vi "Exc time Result.vi"(11 "SubVI":dbl[](array[numeric])) -> (3 "Pos":i32, 5 "Tip":string, 7 "Status":bool)   [LabVIEW 2014]
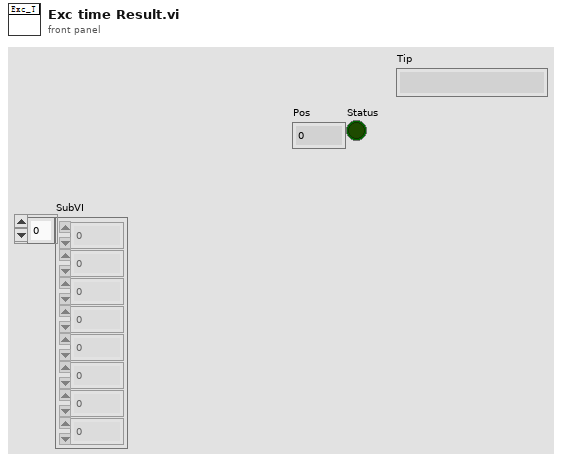
[diagram p1: front panel]
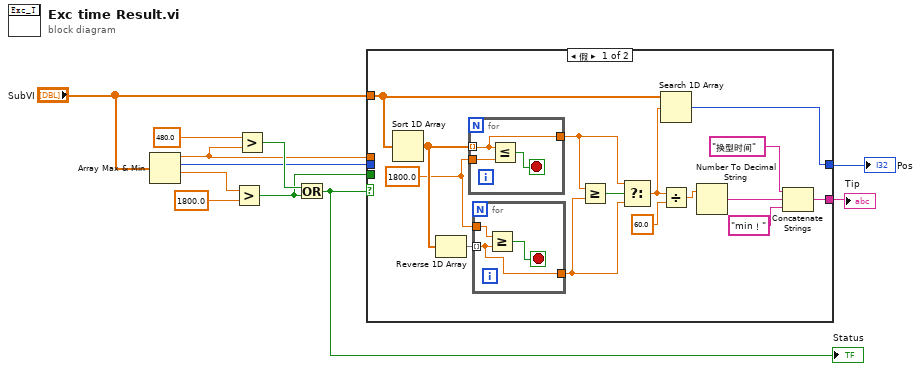
[diagram p0: block diagram]
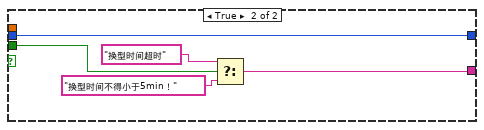
[diagram p2: hidden frame]
diagram:
  n1 = Array Max & Min(array="SubVI") -> (max value=w5:dbl, max index (indices)=w4:i32, min value=w9:dbl)  [unwired: 1 out]
  n2 = Greater?(x=w9, y=1800.0 ("最大值")) -> (0:w3:bool)
  n3 = Greater?(x=480.0 ("最大值"), y=w5) -> (0:w8:bool)
  n4 = Or(x=w8, y=w3) -> (x .or. y?=w7:bool)
  "Status" <- w7
  n5 = case shown="假" w7 {
    tunnel: "SubVI" -> [w16 _]
    tunnel: w5 -> [_ _]
    tunnel: w4 -> [_ w33]
    tunnel: w3 -> [_ w37]
    tunnel: [w26 w34] -> w1
    tunnel: [w15 w33] -> w2
    frame False {
      w20 = 1800.0 ("y")
      n6 = Sort 1D Array(array=w16) -> (sorted array=w22:dbl[])
      n7 = Reverse 1D Array(array=w22) -> (reversed array=w21:dbl[])
      n8 = for {
        tunnel: w22 -> [w30] mode=indexing
        tunnel: w20 -> [w32]
        tunnel: [w30] -> w18
        stop <- w31 stop-if-true
        n9 = Less Or Equal?(x=w30, y=w32) -> (x <= y?=w31:bool)
      }
      n10 = for {
        tunnel: w21 -> [w27] mode=indexing
        tunnel: w20 -> [w29]
        tunnel: [w27] -> w17
        stop <- w28 stop-if-true
        n11 = Greater Or Equal?(x=w29, y=w27) -> (x >= y?=w28:bool)
      }
      n12 = Greater Or Equal?(x=w18, y=w17) -> (x >= y?=w19:bool)
      n13 = Select(t=w18, s=w19, f=w17) -> (s? t:f=w14:dbl)
      n14 = Search 1D Array(1D array=w16, element=w14) -> (index of element=w15:i32)  [unwired: 1 in]
      n15 = Divide(x=w14, y=60.0) -> (x/y=w13:dbl)
      n16 = Number To Decimal String(number=w13) -> (decimal integer string=w24:string)  [unwired: 1 in]
      n17 = Concatenate Strings("换型时间", w24, "min！" ("字符串")) -> (w26:string)
    }
    frame True {
      n18 = Select(t="换型时间超时", s=w37, f="换型时间不得小于5min！") -> (s? t:f=w34:string)
    }
  }
  "Pos" <- w2
  "Tip" <- w1
